vi "ziAutoRange.vi"(8 "Error in":errorcluster, 10 "Path":string, 11 "Handle in":T1 {"Handle" format="0x%08x"; "Conn" format="0x%08x"}) -> (0 "Error out":errorcluster, 1 "Success":bool, 3 "Handle out":T1 {"Handle" format="0x%08x"; "Conn" format="0x%08x"})   [LabVIEW 2019, in "Zurich Instruments LabOne.lvlib"]
doc: "Automatically set the input range of signalinputs/{0,1} to half full level.\n<B>Path</B> can either be sigins/0 or sigins/1"
uses:
  Zurich Instruments LabOne.lvlib
  ziTypeHandle.ctl
  Configure/ziGetValueString.vi
  <vilib>/regexp/Match Regular Expression.xnode
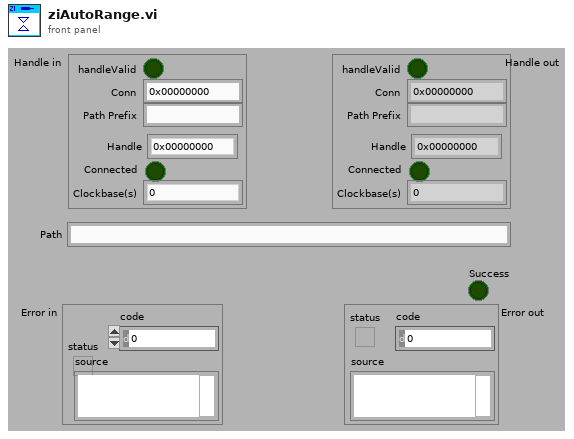
[diagram p1: front panel]
types:
  T1 = typedef "Zurich Instruments LabOne.lvlib/ziTypeHandle.ctl" = cluster{"handleValid":bool, "Conn":u64, "Path Prefix":string, "Handle":u64, "Connected":bool, "Clockbase(s)":dbl}
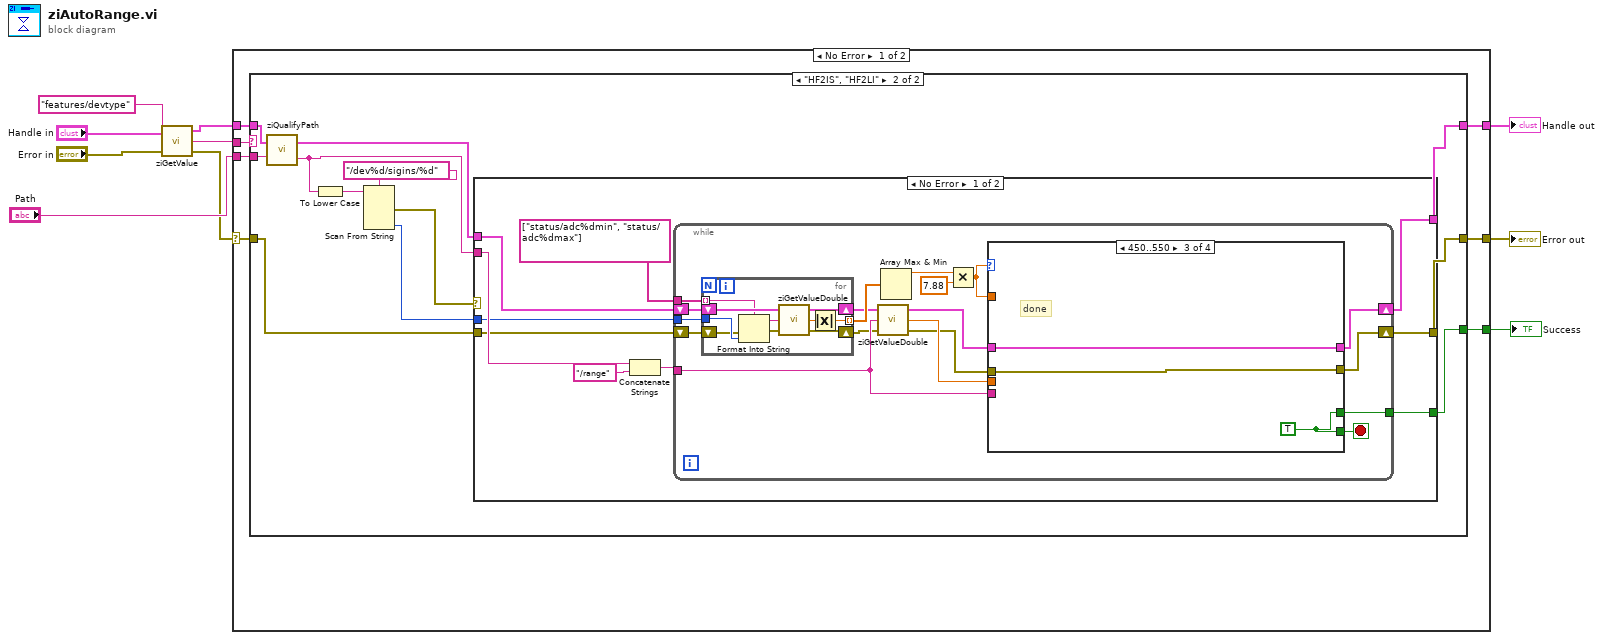
[diagram p0: block diagram]
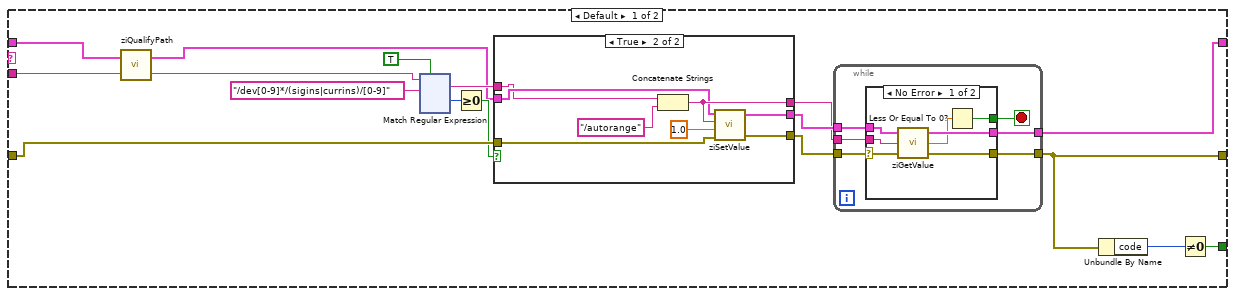
[diagram p2: hidden frame]
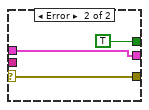
[diagram p3: hidden frame]
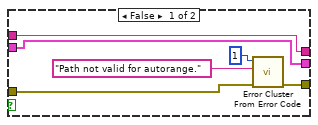
[diagram p4: hidden frame]
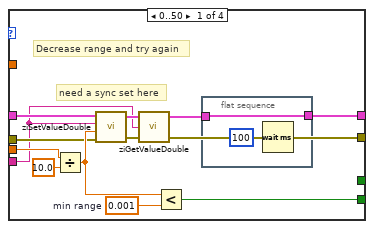
[diagram p5: hidden frame]
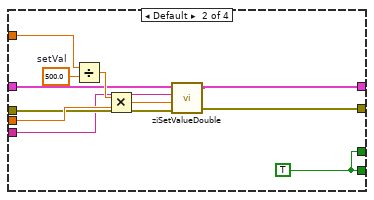
[diagram p6: hidden frame]
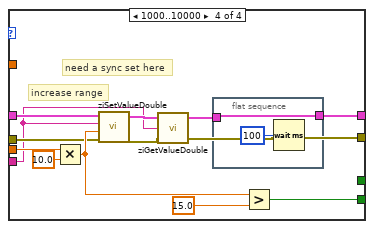
[diagram p7: hidden frame]
diagram:
  n1 = call-poly "ziGetValue.vi"("error in"="Error in", "Path"="features/devtype", "Handle In"="Handle in") -> ("error out"=w2:errorcluster, "Value"=w1:string, "Handle Out"=w3:T1)
  n2 = case shown="No Error" w2 {
    selector: w2 -> [w15 w275]
    tunnel: [w17 w275] -> w10
    tunnel: [w16 w276] -> w9
    tunnel: w3 -> [w13 w276]
    tunnel: "Path" -> [w14 _]
    tunnel: [w12 _] -> w7
    tunnel: w1 -> [w11 _]
    frame No Error {
      n3 = case shown="\"HF2IS\", \"HF2LI\"" w11 {
        tunnel: [w25 w190] -> w17
        tunnel: [w32 w189] -> w16
        tunnel: w15 -> [w34 w188]
        tunnel: w14 -> [w22 w187]
        tunnel: w13 -> [w23 w186]
        tunnel: [w19 w182] -> w12
        frame Default {
          n4 = call "ziQualifyPath.vi"("Path In"=w22, "Handle In"=w23) -> ("Path Out"=w18:string, "Handle Out"=w21:T1)
          n5 = xnode "Match Regular Expression"("input string"=w18, "regular expression"="/dev[0-9]*/(sigins|currins)/[0-9]", "ignore case? (F)"=TRUE) -> ("whole match"=w29:string, "offset past match"=w27:i32)  [unwired: 3 in, 3 out]
          n6 = Greater Or Equal To 0?(x=w27) -> (x >= 0?=w28:bool)
          n7 = case shown="True" w28 {
            tunnel: w34 -> [w168 w178]
            tunnel: w21 -> [w170 w172]
            tunnel: [w170 w175] -> w33
            tunnel: [w169 w174] -> w31
            tunnel: [w167 w173] -> w30
            tunnel: w29 -> [w169 w171]
            frame False {
              n8 = call <vilib>:"Error Cluster From Error Code.vi"("error in (no error)"=w168, "error message (\"\")"="Path not valid for autorange." ("error message (\"\")"), "error code (0)"=1) -> ("error out"=w167:errorcluster)  [unwired: 6 in]
            }
            frame True {
              n9 = Concatenate Strings(w171, "/autorange") -> (w174:string)
              n10 = call-poly "ziSetValue.vi"("Error In"=w178, "Value"=1.0, "Path"=w174, "Handle In"=w172) -> ("Error Out"=w173:errorcluster, "Handle Out"=w175:T1)  [unwired: 1 in]
            }
          }
          n11 = while {
            tunnel: w30 -> [w35]
            tunnel: w33 -> [w40]
            tunnel: [w39] -> w32
            tunnel: w31 -> [w38]
            tunnel: [w36] -> w25
            stop <- w37 stop-if-true
            n12 = case shown="No Error" w35 {
              selector: w35 -> [w41 w49]
              tunnel: w40 -> [w47 w50]
              tunnel: [w46 w50] -> w39
              tunnel: w38 -> [w45 _]
              tunnel: [w44 TRUE] -> w37
              tunnel: [w42 w49] -> w36
              frame No Error {
                n13 = call-poly "ziGetValue.vi"("error in"=w41, "Path"=w45, "Handle in"=w47) -> ("error out"=w42:errorcluster, "Value"=w43:dbl, "Handle out"=w46:T1)
                n14 = Less Or Equal To 0?(x=w43) -> (x <= 0?=w44:bool)
              }
              frame Error {
              }
            }
          }
          n15 = Unbundle By Name(w25) -> ("code"=w20:i32)
          n16 = Not Equal To 0?(x=w20) -> (x != 0?=w19:bool)
        }
        frame "HF2IS", "HF2LI" {
          n17 = call "ziQualifyPath.vi"("Path In"=w187, "Handle In"=w186) -> ("Path Out"=w181:string, "Handle Out"=w185:T1)
          n18 = To Lower Case(string=w181) -> (all lower case string=w180:string)
          n19 = Scan From String(format string="/dev%d/sigins/%d" ("regular expression"), input string=w180) -> (error out=w184:errorcluster, output 2=w179:i32)  [unwired: 5 in, 2 out]
          n20 = case shown="No Error" w184 {
            tunnel: [w197 w274] -> w190
            tunnel: [w198 w273] -> w189
            tunnel: w185 -> [w199 w273]
            tunnel: w188 -> [w191 w274]
            tunnel: w181 -> [w194 _]
            tunnel: w179 -> [w192 _]
            tunnel: [w193 _] -> w182
            frame No Error {
              n21 = Concatenate Strings(w194, "/range") -> (w196:string)
              n22 = while {
                shift-right: [w215] -> w198
                shift-left: w199 -> [w211]
                shift-right: [w214] -> w197
                shift-left: w191 -> [w203]
                tunnel: w196 -> [w206]
                tunnel: string[] ["status/adc%dmin", "status/adc%dmax"] -> [w210]
                tunnel: w192 -> [w202]
                tunnel: [w201] -> w193
                stop <- w213 stop-if-true
                n23 = for {
                  tunnel: w210 -> [w223] mode=indexing
                  tunnel: [w228] -> w218 mode=indexing
                  shift-right: [w227] -> w209
                  shift-left: w211 -> [w226]
                  tunnel: w202 -> [w222]
                  shift-right: [w224] -> w204
                  shift-left: w203 -> [w220]
                  n24 = Format Into String(format string=w223, error in=w220, w222) -> (resulting string=w221:string, error out=w219:errorcluster)  [unwired: 1 in]
                  n25 = call "ziGetValueDouble.vi"("error in"=w219, "Path"=w221, "Handle in"=w226) -> ("error out"=w224:errorcluster, "Value"=w225:dbl, "Handle out"=w227:T1)
                  n26 = Absolute Value(x=w225) -> (abs(x)=w228:dbl)
                }
                n27 = call "ziGetValueDouble.vi"("error in"=w204, "Path"=w206, "Handle in"=w209) -> ("error out"=w205:errorcluster, "Value"=w207:dbl, "Handle out"=w208:T1)
                n28 = Array Max & Min(array=w218) -> (max value=w216:dbl)  [unwired: 3 out]
                n29 = Multiply(x=w216, y=7.88 ("valueD")) -> (x*y=w212:dbl)
                n30 = case shown="450..550" w212 {
                  tunnel: w208 -> [w238 w248 w256 w266]
                  tunnel: w205 -> [w236 w246 w257 w264]
                  tunnel: [w231 w250 w256 w260] -> w215
                  tunnel: [w230 w249 w257 w259] -> w214
                  tunnel: [w229 w244 w255 w267] -> w213
                  tunnel: w207 -> [w241 w254 _ w269]
                  tunnel: w212 -> [_ w252 _ _]
                  tunnel: w206 -> [w234 w245 _ w258]
                  tunnel: [_ w244 w255 _] -> w201
                  frame 0..50 {
                    w239 = 0.001  # min range
                    # "need a sync set here"
                    # "Decrease range and try again"
                    n31 = Divide(x=w241, y=10.0 ("valueD")) -> (x/y=w237:dbl)
                    n32 = call "ziSetValueDouble.vi"("Error In"=w236, "Value"=w237, "Path"=w234, "Handle In"=w238) -> ("Error Out"=w233:errorcluster, "Handle Out"=w235:T1)  [unwired: 1 in]
                    n33 = call "ziGetValueDouble.vi"("error in"=w233, "Path"=w234, "Handle in"=w235) -> ("error out"=w230:errorcluster, "Handle out"=w232:T1)  [unwired: 1 out]
                    n34 = Less?(x=w237, y=w239) -> (x < y?=w229:bool)
                    n35 = flat-sequence {
                      tunnel: w232 -> [w242]
                      tunnel: [w242] -> w231
                      frame #0 {
                        n36 = Wait (ms)(milliseconds to wait=u32 100) -> ()  [unwired: 1 out]
                      }
                    }
                  }
                  frame Default {
                    w251 = 500.0  # setVal
                    w244 = TRUE
                    n37 = Divide(x=w252, y=w251) -> (x/y=w253:dbl)
                    n38 = Multiply(x=w253, y=w254) -> (x*y=w247:dbl)
                    n39 = call "ziSetValueDouble.vi"("Error In"=w246, "Value"=w247, "Path"=w245, "Handle In"=w248) -> ("Error Out"=w249:errorcluster, "Handle Out"=w250:T1)  [unwired: 1 in]
                  }
                  frame 450..550 {
                    w255 = TRUE
                    # "done"
                  }
                  frame 1000..10000 {
                    # "need a sync set here"
                    # "increase range"
                    n40 = Multiply(x=w269, y=10.0 ("valueD")) -> (x*y=w265:dbl)
                    n41 = call "ziSetValueDouble.vi"("Error In"=w264, "Value"=w265, "Path"=w258, "Handle In"=w266) -> ("Error Out"=w262:errorcluster, "Handle Out"=w263:T1)  [unwired: 1 in]
                    n42 = call "ziGetValueDouble.vi"("error in"=w262, "Path"=w258, "Handle in"=w263) -> ("error out"=w259:errorcluster, "Handle out"=w261:T1)  [unwired: 1 out]
                    n43 = flat-sequence {
                      tunnel: w261 -> [w271]
                      tunnel: [w271] -> w260
                      frame #0 {
                        n44 = Wait (ms)(milliseconds to wait=u32 100) -> ()  [unwired: 1 out]
                      }
                    }
                    n45 = Greater?(x=w265, y=15.0 ("valueD")) -> (0:w267:bool)
                  }
                }
              }
            }
            frame Error {
            }
          }
        }
      }
    }
    frame Error {
    }
  }
  "Handle out" <- w9
  "Error out" <- w10
  "Success" <- w7
